vi "校准任务流程.vi"(9 "校准任务":T1[](array[typedef]), 10 "精度":dbl=4.0, 11 "模型":enum32{"线性", "多项式", "折线"}(ring)) -> ()   [LabVIEW 2016, in "斯坦道CODMn新电路板.lvlib"]
uses:
  <userlib>/_OpenG.lib/array/array.llb/Remove Duplicates from 1D Array (U16)__ogtk.vi
panel:
  out "元素":T1
  out "执行列表":T2(ring)
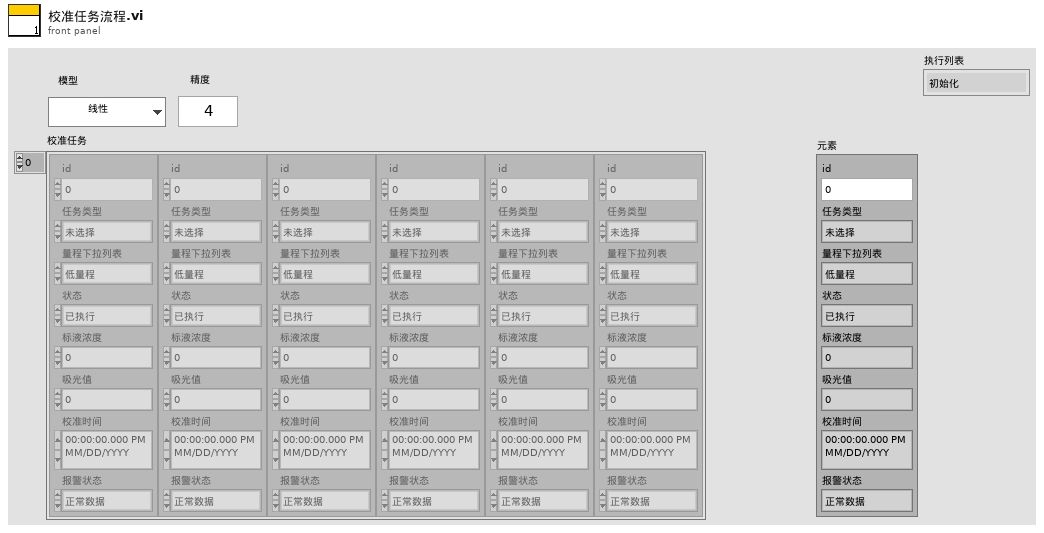
[diagram p1: front panel]
types:
  T1 = typedef "校准任务.ctl" = cluster{"id":u16, "任务类型":enum16{"未选择", "空白校准", "标样校准", "标样核查", "零点核查", "跨度核查"}, "量程下拉列表":enum16{"低量程", "高量程"}, "状态":enum16{"已执行", "待执行", "执行中", "停止"}, "标液浓度":dbl, "吸光值":dbl, "校准时间":timestamp, "报警状态":enum16{"正常数据", "报警数据"}}
  T2 = enum16{"初始化", "解析数据", "判断任务类型", "执行测试任务", "等待测试任务完成", "获取测试数据", "任务结束判定", "计算公式", "结束"}
  T3 = cluster{"时间标识":timestamp, "设备":string, "日志信息":string, "流程参数":string}
  T4 = cluster{"站号":u16, "量程切换":enum32{"H", "L", "AUTO"}, "控制命令":u16, "模式设置":enum16{"待机", "连续模式", "周期模式", "定点模式", "受控模式", "手动模式"}, "测量间隔":u16}
  T5 = cluster{"标液浓度1":dbl, "测量吸光度1":dbl, "样品1启用":bool, "标液浓度2":dbl, "测量吸光度2":dbl, "样品2启用":bool, "标液浓度3":dbl, "测量吸光度3":dbl, "样品3启用":bool, "标液浓度4":dbl, "测量吸光度4":dbl, "样品4启用":bool, "标液浓度5":dbl, "测量吸光度5":dbl, "样品5启用":bool, "模型":enum32{"线性", "多项式", "折线"}, "精度":dbl, "XY图":cluster{"X Values":dbl[], "Y Values":dbl[]}[], "拟合公式":string, "r^2":dbl, "标样一校准时间":timestamp, "标样二校准时间":timestamp, "标样三校准时间":timestamp, "标样四校准时间":timestamp, "标样五校准时间":timestamp, "二次方程":cluster{"x^2":dbl, "K":dbl, "B":dbl}, "标定时间":timestamp, "拟合公式 2":string, "r^2 2":dbl}
  T6 = enum16{"", "水样测量", "标样核查", "零点核查", "跨度核查", "空白测试", "平行样测试", "加标回收", "空白校准", "标样校准"}
  T7 = typedef "报警信息字段定义.ctl" = cluster{"时间":timestamp, "参数":string, "元器件":string, "故障现象":string, "故障分析":string, "state":string, "code":string, "platform_alarm_code":string, "是否上报":string}
  T8 = cluster{"因子编码":u32, "单位":u16, "标样参考值":sgl, "水样数据时间":timestamp, "水样实测值":sgl, "水样数据标识":string, "标样数据时间":timestamp, "标样实测值":sgl, "标样数据标识":string, "空白数据时间":timestamp, "空白实测值":sgl, "空白数据标识":string, "零点核查数据时间":timestamp, "零点核查实测值":sgl, "零点核查数据标识":string, "跨度核查数据时间":timestamp, "跨度核查实测值":sgl, "跨度核查数据标识":string, "加标回收数据时间":timestamp, "加标回收实测值":sgl, "加标回收数据标识":string, "平行样数据时间":timestamp, "平行样实测值":sgl, "平行样数据标识":string, "F0":sgl, "F1":sgl, "F2":sgl, "F3":sgl, "F4":sgl, "F5":sgl, "F6":sgl, "F7":sgl, "温度":sgl, "湿度":sgl, "X值":sgl, "fidrange":u16}
  T9 = cluster{"系统时间":timestamp, "工作状态":u16, "测量模式":enum16{"待机", "连续模式", "周期模式", "定点模式", "受控模式", "手动模式"}, "告警代码":u16, "故障代码":u16, "日志代码":u16, "软件版本":u16, "A":sgl, "B":sgl, "K":sgl, "当前滴定数":sgl, "T":sgl, "H":sgl, "id":u16, "flowid":u16, "量程":u16, "加热实时温度":sgl, "当前ORP值":sgl, "运行时间":sgl, "当前步骤剩余时间":sgl, "结束滴定数":sgl, "注射泵保温温度":sgl, "匹配滴定数X0":u16, "X^2":sgl, "X":sgl, "B 2":sgl, "光值1":sgl, "光值2":sgl, "光值3":sgl, "光值4":sgl, "光值5":sgl, "光值6":sgl, "光值7":sgl, "光值8":sgl}
  T10 = enum16{"未选择", "空白校准", "标样校准", "标样核查", "零点核查", "跨度核查"}
  T11 = cluster{"标液浓度1":dbl, "测量吸光度1":dbl, "样品1启用":bool, "标液浓度2":dbl, "测量吸光度2":dbl, "样品2启用":bool, "标液浓度3":dbl, "测量吸光度3":dbl, "样品3启用":bool, "标液浓度4":dbl, "测量吸光度4":dbl, "样品4启用":bool, "标液浓度5":dbl, "测量吸光度5":dbl, "样品5启用":bool, "模型":enum32{"线性", "多项式", "折线"}, "精度":dbl, "XY图":cluster{"X Values":dbl[], "Y Values":dbl[]}[], "拟合公式":string, "r^2":dbl, "标样一校准时间":timestamp, "标样二校准时间":timestamp, "标样三校准时间":timestamp, "标样四校准时间":timestamp, "标样五校准时间":timestamp, "二次方程":cluster{"c":dbl, "x":dbl, "x^2":dbl}, "标定时间":timestamp, "拟合公式 2":string, "r^2 2":dbl}[][]
  T12 = cluster{"标液浓度1":dbl, "测量吸光度1":dbl, "样品1启用":bool, "标液浓度2":dbl, "测量吸光度2":dbl, "样品2启用":bool, "标液浓度3":dbl, "测量吸光度3":dbl, "样品3启用":bool, "标液浓度4":dbl, "测量吸光度4":dbl, "样品4启用":bool, "标液浓度5":dbl, "测量吸光度5":dbl, "样品5启用":bool, "模型":enum32{"线性", "多项式", "折线"}, "精度":dbl, "XY图":cluster{"X Values":dbl[], "Y Values":dbl[]}[], "拟合公式":string, "r^2":dbl, "标样一校准时间":timestamp, "标样二校准时间":timestamp, "标样三校准时间":timestamp, "标样四校准时间":timestamp, "标样五校准时间":timestamp, "二次方程":cluster{"c":dbl, "x":dbl, "x^2":dbl}, "标定时间":timestamp, "拟合公式 2":string, "r^2 2":dbl}
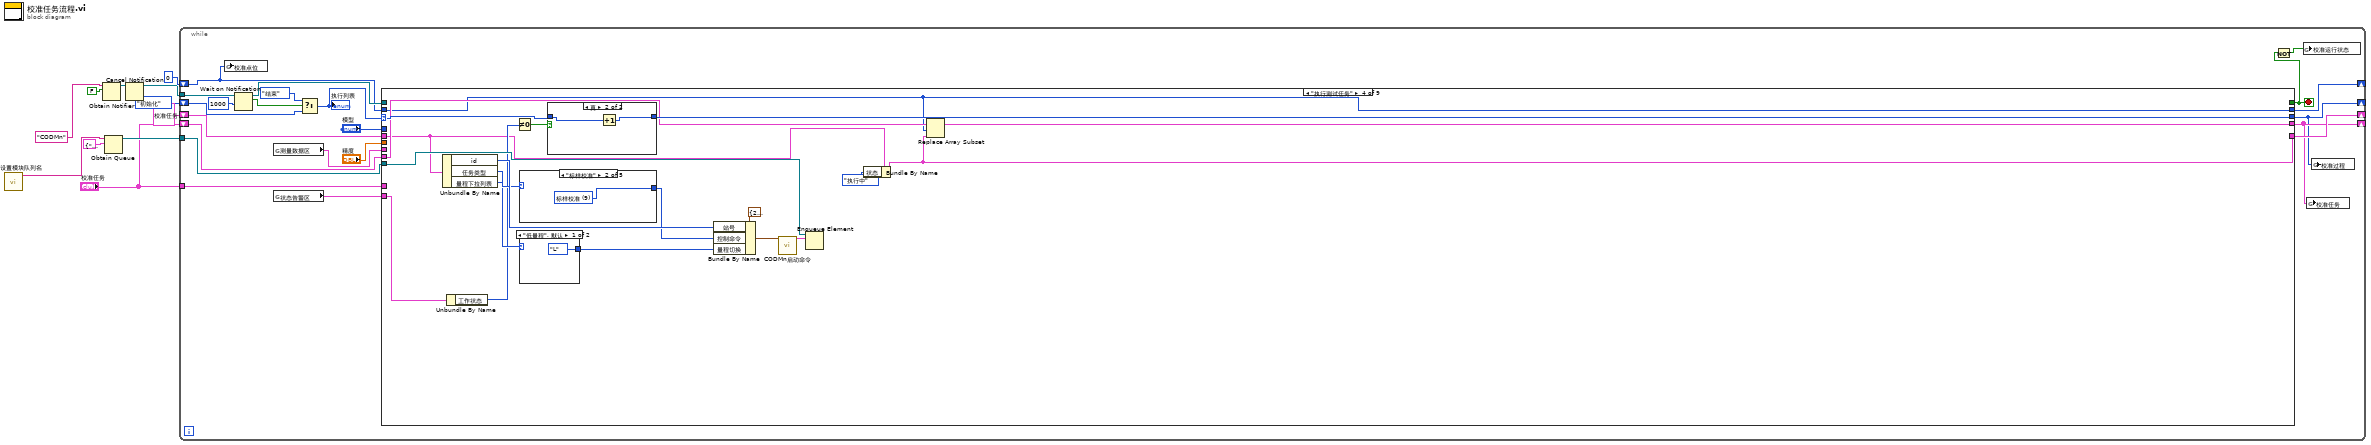
[diagram p0: block diagram]
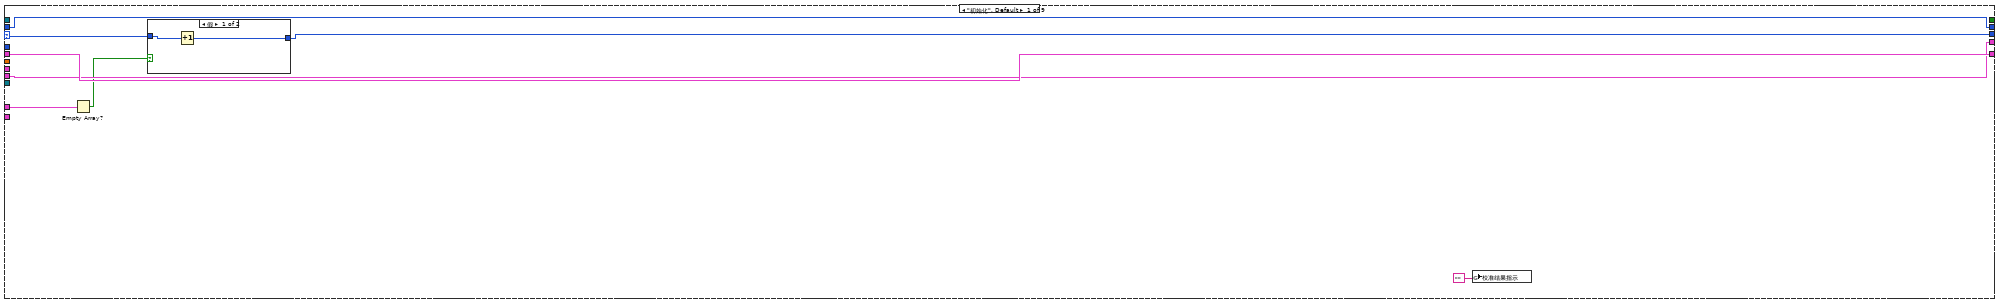
[diagram p2: hidden frame]
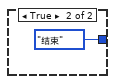
[diagram p3: hidden frame]
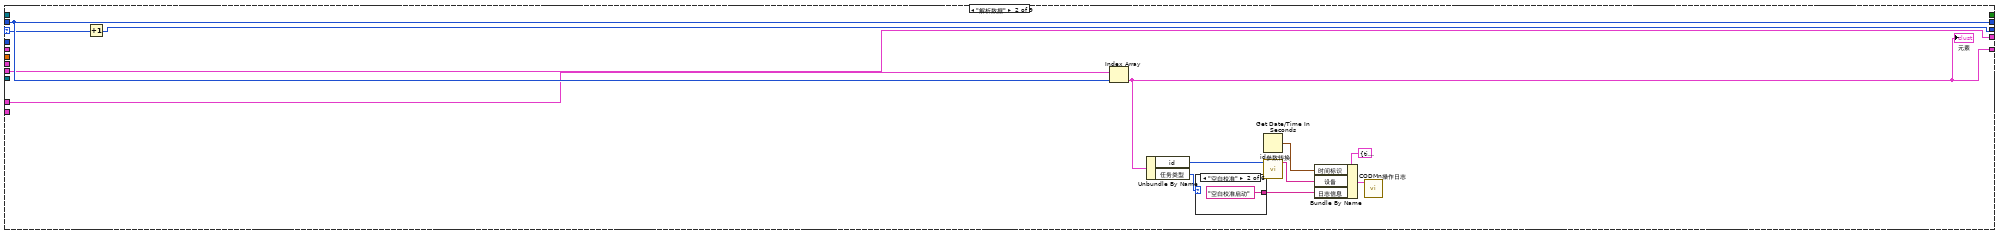
[diagram p4: hidden frame]
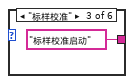
[diagram p6: hidden frame]
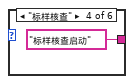
[diagram p7: hidden frame]
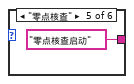
[diagram p8: hidden frame]
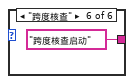
[diagram p9: hidden frame]
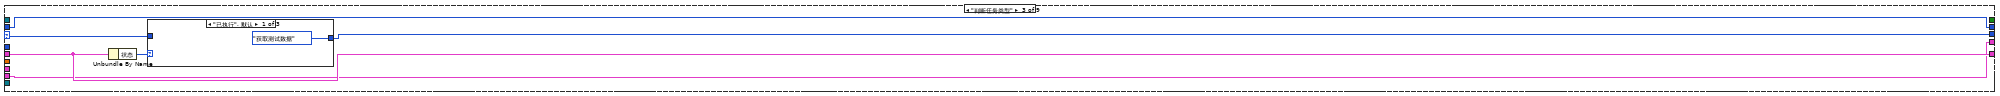
[diagram p10: hidden frame]
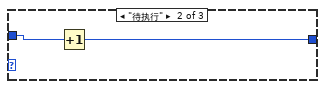
[diagram p11: hidden frame]
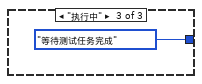
[diagram p12: hidden frame]
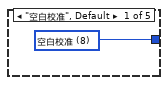
[diagram p14: hidden frame]
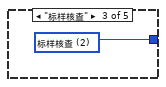
[diagram p15: hidden frame]
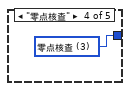
[diagram p16: hidden frame]
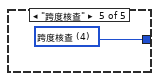
[diagram p17: hidden frame]
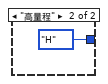
[diagram p18: hidden frame]
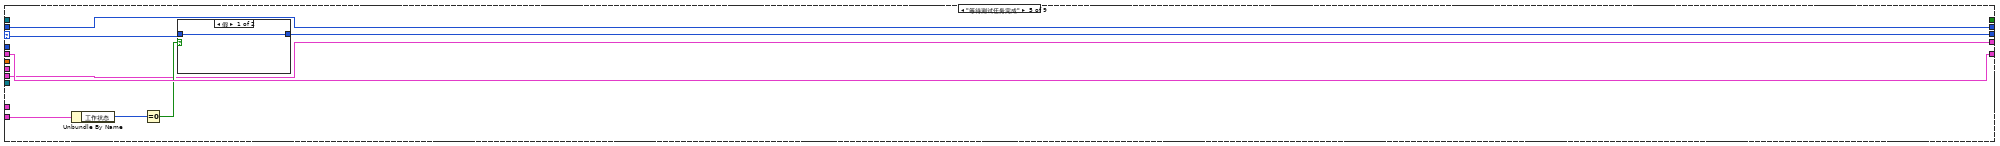
[diagram p19: hidden frame]
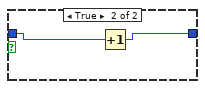
[diagram p20: hidden frame]
diagram:
  n1 = call "设置模块队列名.vi"() -> ("Msg"=w1:string)  [unwired: 11 in]
  n2 = Obtain Notifier(name (unnamed)="CODMn" ("名称（未命名）"), notification data type=FALSE) -> (notifier out=w6:refnum<notifier>)  [unwired: 2 in, 2 out]
  n3 = Obtain Queue(name (unnamed)=w1, element data type=cluster{"命令":string, "data":variant} {"命令"="", "data"=variant}) -> (queue out=w7:refnum<queue>)  [unwired: 3 in, 2 out]
  n4 = Cancel Notification(0:w6) -> (8:w5:refnum<notifier>)  [unwired: 1 in, 2 out]
  n5 = while {
    shift-right: [w13] -> _
    shift-left: 0 -> [w15]
    shift-right: [w33] -> _
    shift-left: T1 {"id"=0, "任务类型"=enum."未选择", "量程下拉列表"=enum."低量程", "状态"=enum."待执行", "标液浓度"=0.0, "吸光值"=0.0, "校准时间"=timestamp(0 s since 1904-01-01), "报警状态"=enum."正常数据"} ("校准任务") -> [w32]
    shift-right: [w12] -> _
    shift-left: T2."初始化" ("执行列表") -> [w21]
    tunnel: w7 -> [w31]
    tunnel: w5 -> [w30]
    tunnel: "校准任务" -> [w27]
    shift-right: [w14] -> _
    shift-left: "校准任务" -> [w26]
    stop <- w16 stop-if-true
    n6 = global write "VARCODMn全局变量.vi" "校准点位"(w15) -> ()
    n7 = Wait on Notification(notifier=w30, timeout in ms (-1)=1000 ("超时毫秒(-1)")) -> (notifier out=w23:refnum<notifier>, notification=w22:bool)  [unwired: 2 in, 2 out]
    n8 = global read "VARCODMn全局变量.vi" "测量数据区"() -> (w28:T8)
    n9 = global read "VARCODMn全局变量.vi" "状态告警区"() -> (w29:T9)
    n10 = Select(t=T2."结束", s=w22, f=w21) -> (s? t:f=w20:T2)
    "执行列表" <- w20
    n11 = case shown="\"执行测试任务\"" w20 {
      selector: w20 -> [w39 w56 w65 w83 w106 w124 w167 w181 w375]
      tunnel: w15 -> [w40 w57 w67 w79 w109 w115 w168 w179 w373]
      tunnel: [w41 w48 w68 w76 w110 w119 w169 w178 w374] -> w33
      tunnel: w32 -> [w41 _ w68 w78 w110 w119 w169 w178 w374]
      tunnel: [w40 w57 w67 w79 w109 w115 w164 w179 w373] -> w13
      tunnel: [_ _ _ _ _ _ _ _ TRUE] -> w16
      tunnel: [w38 w55 w64 w82 w104 w123 w166 w180 w375] -> w12
      tunnel: w31 -> [_ _ _ w91 _ _ _ _ w370]
      tunnel: w23 -> [_ _ _ _ _ _ _ _ w369]
      tunnel: w29 -> [_ _ _ w86 w108 w114 _ _ _]
      tunnel: w28 -> [_ _ _ _ _ w126 _ _ _]
      tunnel: w27 -> [w36 w54 _ _ _ _ w165 _ _]
      tunnel: [w35 w53 w63 w80 w103 w121 w161 w177 w371] -> w14
      tunnel: w26 -> [w35 w53 w63 w81 w103 w120 w161 w177 w371]
      tunnel: "模型" -> [_ _ _ _ _ _ _ w176 _]
      tunnel: "精度" -> [_ _ _ _ _ _ _ w175 _]
      frame "初始化", Default {
        n12 = Empty Array?(array=w36) -> (empty?=w34:bool)
        n13 = case shown="假" w34 {
          tunnel: w39 -> [w43 _]
          tunnel: [w42 T2."结束"] -> w38
          frame False {
            n14 = Increment(x=w43) -> (x+1=w42:T2)
          }
          frame True {
          }
        }
        n15 = global write "VARCODMn全局变量.vi" "校准结果指示"("") -> ()
      }
      frame "解析数据" {
        n16 = Increment(x=w56) -> (x+1=w55:T2)
        n17 = Index Array(array=w54, index=w57) -> (element=w48:T1)
        "元素" <- w48
        n18 = Unbundle By Name(w48) -> ("id"=w47:u16, "任务类型"=w46:T10)
        n19 = case shown="\"空白校准\"" w46 {
          tunnel: [_ "空白校准启动" "标样校准启动" "标样核查启动" "零点核查启动" "跨度核查启动"] -> w45
          frame "未选择", Default {
          }
          frame "空白校准" {
          }
          frame "标样校准" {
          }
          frame "标样核查" {
          }
          frame "零点核查" {
          }
          frame "跨度核查" {
          }
        }
        n20 = Get Date/Time In Seconds() -> (seconds since 1Jan1904=w52:timestamp)
        n21 = call "id参数转换.vi"("id"=w47) -> ("table输出"=w49:string)  [unwired: 10 in]
        n22 = Bundle By Name(cluster=T3 {"时间标识"=timestamp(0 s since 1904-01-01), "设备"="", "日志信息"="", "流程参数"=""} ("data in"), "时间标识"=w52, "设备"=w49, "日志信息"=w45) -> (w51:T3)
        n23 = call "CODMn操作日志.vi"("data in"=w51) -> ()  [unwired: 11 in]
      }
      frame "判断任务类型" {
        n24 = Unbundle By Name(w68) -> ("状态"=w66:enum16{"已执行", "待执行", "执行中", "停止"})
        n25 = case shown="\"已执行\", 默认" w66 {
          tunnel: w65 -> [_ w71 _]
          tunnel: [T2."获取测试数据" w70 T2."等待测试任务完成"] -> w64
          frame "已执行", Default {
          }
          frame "待执行" {
            n26 = Increment(x=w71) -> (x+1=w70:T2)
          }
          frame "执行中" {
          }
        }
      }
      frame "执行测试任务" {
        n27 = Unbundle By Name(w78) -> ("id"=w90:u16, "任务类型"=w89:T10, "量程下拉列表"=w88:enum16{"低量程", "高量程"})
        n28 = Unbundle By Name(w86) -> ("工作状态"=w85:u16)
        n29 = Not Equal To 0?(x=w85) -> (x != 0?=w84:bool)
        n30 = case shown="\"标样校准\"" w89 {
          tunnel: [w96 w97 w98 w99 w100] -> w73
          frame "空白校准", Default {
            w96 = u16 8 items=["启动测量"=1, "标样核查"=2, "零点核查"=3, "跨度核查"=4, "空白测试"=5, "平行样测试"=6, "加标回收"=7, "空白校准"=8, "标样校准"=9, "初始化（清洗）"=10, "停止测试"=11, "仪器重启"=12, "校时"=13, "模式设置"=14, "测量间隔设置"=15, "调试"=22, "填充管路"=30, "清洗管路"=31, "清洗反应杯"=32] ("控制命令")
          }
          frame "标样校准" {
            w97 = u16 9 items=["启动测量"=1, "标样核查"=2, "零点核查"=3, "跨度核查"=4, "空白测试"=5, "平行样测试"=6, "加标回收"=7, "空白校准"=8, "标样校准"=9, "初始化（清洗）"=10, "停止测试"=11, "仪器重启"=12, "校时"=13, "模式设置"=14, "测量间隔设置"=15, "调试"=22, "填充管路"=30, "清洗管路"=31, "清洗反应杯"=32] ("控制命令")
          }
          frame "标样核查" {
            w98 = u16 2 items=["启动测量"=1, "标样核查"=2, "零点核查"=3, "跨度核查"=4, "空白测试"=5, "平行样测试"=6, "加标回收"=7, "空白校准"=8, "标样校准"=9, "初始化（清洗）"=10, "停止测试"=11, "仪器重启"=12, "校时"=13, "模式设置"=14, "测量间隔设置"=15, "调试"=22, "填充管路"=30, "清洗管路"=31, "清洗反应杯"=32] ("控制命令")
          }
          frame "零点核查" {
            w99 = u16 3 items=["启动测量"=1, "标样核查"=2, "零点核查"=3, "跨度核查"=4, "空白测试"=5, "平行样测试"=6, "加标回收"=7, "空白校准"=8, "标样校准"=9, "初始化（清洗）"=10, "停止测试"=11, "仪器重启"=12, "校时"=13, "模式设置"=14, "测量间隔设置"=15, "调试"=22, "填充管路"=30, "清洗管路"=31, "清洗反应杯"=32] ("控制命令")
          }
          frame "跨度核查" {
            w100 = u16 4 items=["启动测量"=1, "标样核查"=2, "零点核查"=3, "跨度核查"=4, "空白测试"=5, "平行样测试"=6, "加标回收"=7, "空白校准"=8, "标样校准"=9, "初始化（清洗）"=10, "停止测试"=11, "仪器重启"=12, "校时"=13, "模式设置"=14, "测量间隔设置"=15, "调试"=22, "填充管路"=30, "清洗管路"=31, "清洗反应杯"=32] ("控制命令")
          }
        }
        n31 = case shown="\"低量程\", 默认" w88 {
          tunnel: [enum32{"H", "L", "AUTO"}."L" ("量程切换") enum32{"H", "L", "AUTO"}."H" ("量程切换")] -> w87
          frame "低量程", Default {
          }
          frame "高量程" {
          }
        }
        n32 = case shown="真" w84 {
          tunnel: w83 -> [w93 w95]
          tunnel: [w93 w94] -> w82
          frame False {
          }
          frame True {
            n33 = Increment(x=w95) -> (x+1=w94:T2)
          }
        }
        n34 = Bundle By Name(cluster=T4 {"站号"=21, "量程切换"=enum."AUTO", "控制命令"=0, "模式设置"=enum."待机", "测量间隔"=0} ("参数"), "站号"=w90, "控制命令"=w73, "量程切换"=w87) -> (w74:T4)
        n35 = call "CODMn启动命令.vi"("参数"=w74) -> ("启动命令"=w92:cluster{"命令":string, "data":variant})  [unwired: 10 in]
        n36 = Enqueue Element(queue=w91, element=w92) -> ()  [unwired: 2 in, 3 out]
        n37 = Bundle By Name(cluster=w78, "状态"=enum16{"已执行", "待执行", "执行中", "停止"}."执行中") -> (w76:T1)
        n38 = Replace Array Subset(array=w81, new element=w76, index=w79) -> (w80:T1[])
      }
      frame "等待测试任务完成" {
        n39 = Unbundle By Name(w108) -> ("工作状态"=w107:u16)
        n40 = Equal To 0?(x=w107) -> (x = 0?=w105:bool)
        n41 = case shown="假" w105 {
          tunnel: w106 -> [w111 w113]
          tunnel: [w111 w112] -> w104
          frame False {
          }
          frame True {
            n42 = Increment(x=w113) -> (x+1=w112:T2)
          }
        }
      }
      frame "获取测试数据" {
        n43 = Unbundle By Name(w119) -> ("任务类型"=w125:T10, "状态"=w118:enum16{"已执行", "待执行", "执行中", "停止"})
        n44 = Increment(x=w124) -> (x+1=w123:T2)
        n45 = case shown="\"待执行\", 默认" w118 {
          tunnel: w126 -> [_ w135]
          tunnel: w125 -> [_ w134]
          tunnel: [w127 w131] -> w122
          tunnel: w119 -> [w127 w130]
          tunnel: w114 -> [_ w129]
          frame "已执行" {
          }
          frame "待执行", Default {
            n46 = case shown="\"跨度核查\"" w134 {
              tunnel: w135 -> [w140 w145 w150 w155 w160]
              tunnel: [w139 w144 w149 w154 w159] -> w132
              tunnel: [w137 w142 w147 w152 w157] -> w133
              tunnel: w129 -> [w138 w143 w148 w153 w158]
              tunnel: [w136 w141 w146 w151 w156] -> w128
              frame "空白校准", Default {
                n47 = Unbundle By Name(w138) -> ("结束滴定数"=w137:sgl, "告警代码"=w136:u16)
                n48 = Unbundle By Name(w140) -> ("空白数据时间"=w139:timestamp)
              }
              frame "标样校准" {
                n49 = Unbundle By Name(w143) -> ("结束滴定数"=w142:sgl, "告警代码"=w141:u16)
                n50 = Unbundle By Name(w145) -> ("标样数据时间"=w144:timestamp)
              }
              frame "标样核查" {
                n51 = Unbundle By Name(w148) -> ("结束滴定数"=w147:sgl, "告警代码"=w146:u16)
                n52 = Unbundle By Name(w150) -> ("标样数据时间"=w149:timestamp)
              }
              frame "零点核查" {
                n53 = Unbundle By Name(w155) -> ("零点核查数据时间"=w154:timestamp)
                n54 = Unbundle By Name(w153) -> ("结束滴定数"=w152:sgl, "告警代码"=w151:u16)
              }
              frame "跨度核查" {
                n55 = Unbundle By Name(w158) -> ("结束滴定数"=w157:sgl, "告警代码"=w156:u16)
                n56 = Unbundle By Name(w160) -> ("跨度核查数据时间"=w159:timestamp)
              }
            }
            n57 = Bundle By Name(cluster=w130, "校准时间"=w132, "吸光值"=w133, "报警状态"=w128) -> (w131:T1)
          }
        }
        n58 = Bundle By Name(cluster=w122, "状态"=enum16{"已执行", "待执行", "执行中", "停止"}."已执行") -> (w116:T1)
        n59 = Replace Array Subset(array=w120, new element=w116, index=w115) -> (w121:T1[])
      }
      frame "任务结束判定" {
        n60 = Array Size(array=w165) -> (size(s)=w163:i32)
        n61 = Increment(x=w168) -> (x+1=w164:i32)
        n62 = Greater Or Equal?(x=w164, y=w163) -> (x >= y?=w162:bool)
        n63 = case shown="假" w162 {
          tunnel: w167 -> [_ w173]
          tunnel: [T2."解析数据" w172] -> w166
          frame False {
            n64 = Wait (ms)(milliseconds to wait=u32 3000 ("等待时间（毫秒）")) -> ()  [unwired: 1 out]
          }
          frame True {
            n65 = Increment(x=w173) -> (x+1=w172:T2)
          }
        }
      }
      frame "计算公式" {
        n66 = flat-sequence {
          tunnel: w181 -> [w188]
          tunnel: w177 -> [w184]
          tunnel: w176 -> [w183]
          tunnel: w175 -> [w182]
          tunnel: [w187] -> w174
          tunnel: [w368] -> w180
          tunnel: w174 -> [w368]
          frame #0 {
            n67 = for {
              tunnel: w184 -> [w367] mode=indexing
              tunnel: [w366] -> w186 mode=indexing
              n68 = Unbundle By Name(w367) -> ("id"=w366:u16)
            }
            n69 = Increment(x=w188) -> (x+1=w187:T2)
            n70 = call-poly <userlib>:"Remove Duplicates from 1D Array__ogtk.vi"("Input Array"=w186) -> ("Output Array"=w185:u16[])  [unwired: 1 out]
            n71 = for {
              tunnel: w185 -> [w201] mode=indexing
              tunnel: w184 -> [w203]
              tunnel: w183 -> [w200]
              tunnel: w182 -> [w199]
              n72 = for {
                tunnel: w203 -> [w363] mode=indexing
                tunnel: w201 -> [w365]
                tunnel: [w363] -> w202 mode=indexing if=w364
                n73 = Unbundle By Name(w363) -> ("id"=w362:u16)
                n74 = Equal?(x=w362, y=w365) -> (x = y?=w364:bool)
              }
              n75 = flat-sequence {
                tunnel: w202 -> [w216]
                tunnel: w201 -> [w211]
                tunnel: w200 -> [w215]
                tunnel: w199 -> [w214]
                tunnel: T5 {"标液浓度1"=0.0, "测量吸光度1"=0.0, "样品1启用"=FALSE, "标液浓度2"=0.0, "测量吸光度2"=0.0, "样品2启用"=FALSE, "标液浓度3"=0.0, "测量吸光度3"=0.0, "样品3启用"=FALSE, "标液浓度4"=0.0, "测量吸光度4"=0.0, "样品4启用"=FALSE, "标液浓度5"=0.0, "测量吸光度5"=0.0, "样品5启用"=FALSE, "模型"=enum."线性", "精度"=4.0, "XY图"=[], "拟合公式"="", "r^2"=0.0, "标样一校准时间"=timestamp(0 s since 1904-01-01), "标样二校准时间"=timestamp(0 s since 1904-01-01), "标样三校准时间"=timestamp(0 s since 1904-01-01), "标样四校准时间"=timestamp(0 s since 1904-01-01), "标样五校准时间"=timestamp(0 s since 1904-01-01), "二次方程"={"x^2"=0.0, "K"=0.0, "B"=0.0}, "标定时间"=timestamp(0 s since 1904-01-01), "拟合公式 2"="", "r^2 2"=0.0} ("曲线模型") -> [w213]
                tunnel: [w212] -> w198
                tunnel: [w211] -> w197
                tunnel: [w210] -> w196
                tunnel: [w209] -> w194
                tunnel: cluster{"x^2":dbl, "K":dbl, "B":dbl} {"x^2"=0.0, "K"=0.0, "B"=0.0} ("二次方程 2") -> [w208]
                tunnel: [w207] -> w193
                tunnel: 0.0 ("公式切换阈值滴定数(0~9999)") -> [w206]
                tunnel: [w205] -> w191
                tunnel: TRUE -> [w204]
                tunnel: w198 -> [w290]
                tunnel: w197 -> [w292]
                tunnel: w196 -> [w291]
                tunnel: w194 -> [w288]
                tunnel: w193 -> [w287]
                tunnel: w191 -> [w282]
                frame #0 {
                  n76 = for {
                    tunnel: w216 -> [w238] mode=indexing
                    tunnel: w211 -> [_]
                    tunnel: w215 -> [w235]
                    tunnel: w214 -> [w234]
                    shift-right: [w226] -> w212
                    shift-left: w213 -> [w233]
                    tunnel: [w224] -> w210
                    shift-right: [w223] -> w209
                    shift-left: w208 -> [_]
                    shift-right: [w222] -> w207
                    shift-left: w206 -> [_]
                    shift-right: [w219] -> w205
                    shift-left: w204 -> [w217]
                    n77 = Unbundle By Name(w238) -> ("标液浓度"=w237:dbl, "吸光值"=w236:dbl, "任务类型"=w225:T10, "量程下拉列表"=w224:enum16{"低量程", "高量程"}, "校准时间"=w232:timestamp, "报警状态"=w220:enum16{"正常数据", "报警数据"})
                    n78 = Get Date/Time In Seconds() -> (seconds since 1Jan1904=w228:timestamp)
                    n79 = Greater Than 0?(x=w220) -> (x > 0?=w218:bool)
                    n80 = case shown="假" w218 {
                      tunnel: [w239 FALSE] -> w219
                      tunnel: w217 -> [w239 _]
                      frame False {
                      }
                      frame True {
                      }
                    }
                    n81 = case shown="\"空白校准\"" w225 {
                      tunnel: w237 -> [_ w249 w257 w265 w273 w281]
                      tunnel: w236 -> [_ w248 w250 w264 w272 w280]
                      tunnel: w235 -> [_ w247 w256 w263 w271 w279]
                      tunnel: w234 -> [_ w246 w255 w262 w270 w278]
                      tunnel: w233 -> [w241 w244 w253 w260 w268 w276]
                      tunnel: [w241 w242 w252 w259 w267 w275] -> w231
                      tunnel: w232 -> [_ w243 w251 w258 w266 w274]
                      frame "未选择", Default {
                        (unwired) T6."" ("测量模式")
                      }
                      frame "空白校准" {
                        n82 = Bundle By Name(cluster=w244, "标液浓度1"=w249, "测量吸光度1"=w248, "模型"=w247, "精度"=w246, "样品1启用"=TRUE, "标样一校准时间"=w243) -> (w242:T5)
                      }
                      frame "标样校准" {
                        (unwired) T6."标样校准" ("测量模式")
                        n83 = Bundle By Name(cluster=w253, "标液浓度2"=w257, "测量吸光度2"=w250, "模型"=w256, "精度"=w255, "样品2启用"=TRUE ("样品1启用"), "标样二校准时间"=w251) -> (w252:T5)
                      }
                      frame "标样核查" {
                        (unwired) T6."标样核查" ("测量模式")
                        n84 = Bundle By Name(cluster=w260, "标液浓度3"=w265, "测量吸光度3"=w264, "模型"=w263, "精度"=w262, "样品3启用"=TRUE ("样品1启用"), "标样三校准时间"=w258) -> (w259:T5)
                      }
                      frame "零点核查" {
                        (unwired) T6."零点核查" ("测量模式")
                        n85 = Bundle By Name(cluster=w268, "标液浓度4"=w273, "测量吸光度4"=w272, "模型"=w271, "精度"=w270, "样品4启用"=TRUE ("样品1启用"), "标样四校准时间"=w266) -> (w267:T5)
                      }
                      frame "跨度核查" {
                        (unwired) T6."跨度核查" ("测量模式")
                        n86 = Bundle By Name(cluster=w276, "标液浓度5"=w281, "测量吸光度5"=w280, "模型"=w279, "精度"=w278, "样品5启用"=TRUE ("样品1启用"), "标样五校准时间"=w274) -> (w275:T5)
                      }
                    }
                    n87 = global read "校准数据全局变量.vi" "CODMn曲线模型"() -> (w230:T11)
                    n88 = call "曲线模型计算.vi"("曲线模型"=w231) -> ("公式切换阈值滴定数(0~9999)"=w222:dbl, "二次方程 2"=w223:cluster{"x^2":dbl, "K":dbl, "B":dbl}, "输出簇"=w227:T12)  [unwired: 8 in]
                    n89 = Bundle By Name(cluster=w227, "标定时间"=w228) -> (w226:T12)
                    n90 = Replace Array Subset(array=w230, new element=w226, index (row)=T6."水样测量" ("测量模式"), index (col)=w224) -> (w229:T11)
                    n91 = global write "校准数据全局变量.vi" "CODMn曲线模型"(w229) -> ()
                  }
                }
                frame #1 {
                  n92 = Unbundle By Name(w290) -> ("r^2"=w285:dbl, "r^2 2"=w284:dbl, "二次方程"=w293:cluster{"x^2":dbl, "K":dbl, "B":dbl}, "模型"=w286:enum32{"线性", "多项式", "折线"})
                  n93 = case shown="\"线性\", 默认" w286 {
                    tunnel: w285 -> [w298 w302]
                    tunnel: w284 -> [_ w303]
                    tunnel: [w295 w304] -> w283
                    tunnel: w282 -> [w294 w300]
                    frame "线性", Default {
                      n94 = global read "CODMn断电保存全局变量.vi" "校准条件"() -> (w299:cluster{"线性相关系数":dbl})
                      n95 = Unbundle By Name(w299) -> ("线性相关系数"=w297:dbl)
                      n96 = Greater Or Equal?(x=w298, y=w297) -> (x >= y?=w296:bool)
                      n97 = And(x=w294, y=w296) -> (x .and. y?=w295:bool)
                    }
                    frame "折线" {
                      n98 = global read "CODMn断电保存全局变量.vi" "校准条件"() -> (w307:cluster{"线性相关系数":dbl})
                      n99 = Unbundle By Name(w307) -> ("线性相关系数"=w301:dbl)
                      n100 = Greater Or Equal?(x=w302, y=w301) -> (x >= y?=w306:bool)
                      n101 = Greater Or Equal?(x=w303, y=w301) -> (x >= y?=w305:bool)
                      n102 = Compound Arithmetic op=AND ("复合运算")(w306, w305, w300) -> (w304:bool)
                    }
                  }
                  n103 = case shown="真" w283 {
                    tunnel: w293 -> [_ w332]
                    tunnel: w292 -> [w313 _]
                    tunnel: w291 -> [_ w321]
                    tunnel: w290 -> [_ w331]
                    tunnel: [w308 w330] -> w289
                    tunnel: w288 -> [_ w329]
                    tunnel: w287 -> [_ w320]
                    tunnel: w282 -> [w310 _]
                    frame False {
                      n104 = case shown="假" w310 {
                        tunnel: ["有故障数据" ("格式字符串") "校准条件未满足" ("格式字符串")] -> w309
                        frame False {
                        }
                        frame True {
                        }
                      }
                      n105 = call "id参数转换.vi"("id"=w313) -> ("table输出"=w312:string)  [unwired: 10 in]
                      n106 = Get Date/Time In Seconds() -> (seconds since 1Jan1904=w316:timestamp)
                      n107 = Format Into String(format string="校准失败，%s" ("格式字符串"), w309) -> (resulting string=w308:string)  [unwired: 2 in, 1 out]
                      n108 = Bundle By Name(cluster=T3 {"时间标识"=timestamp(0 s since 1904-01-01), "设备"="", "日志信息"="", "流程参数"=""} ("data in"), "时间标识"=w316, "设备"=w312, "日志信息"=w308) -> (w315:T3)
                      n109 = call "CODMn操作日志.vi"("data in"=w315) -> ()  [unwired: 11 in]
                    }
                    frame True {
                      n110 = Unbundle By Name(w329) -> ("x^2"=w325:dbl, "K"=w324:dbl, "B"=w323:dbl)
                      n111 = Unbundle By Name(w332) -> ("x^2"=w334:dbl, "K"=w335:dbl, "B"=w336:dbl)
                      n112 = Bundle By Name(cluster=cluster{"X^2":dbl, "X":dbl, "b":dbl} {"X^2"=0.0, "X"=0.0, "b"=0.0} ("公式"), "X^2"=w334, "X"=w335, "b"=w336) -> (w327:cluster{"X^2":dbl, "X":dbl, "b":dbl})
                      n113 = Bundle By Name(cluster=cluster{"X^2":dbl, "X":dbl, "b":dbl} {"X^2"=0.0, "X"=0.0, "b"=0.0} ("公式"), "X^2"=w325, "X"=w324, "b"=w323) -> (w322:cluster{"X^2":dbl, "X":dbl, "b":dbl})
                      n114 = for {
                        N: 7 -> [_]
                        tunnel: w327 -> [w347]
                        tunnel: [w345] -> w319
                        tunnel: w322 -> [w344]
                        tunnel: w320 -> [w343]
                        tunnel: w321 -> [w341]
                        i -> [w338]
                        w342 = enum16{"CODMn"}."CODMn" ("测量参数")
                        n115 = case shown="\"高量程\"" w341 {
                          tunnel: [enum16{"低量程1", "低量程2", "高量程1", "高量程2"}."低量程1" ("量程") enum16{"低量程1", "低量程2", "高量程1", "高量程2"}."高量程1" ("量程")] -> w340
                          tunnel: [enum16{"低量程1", "低量程2", "高量程1", "高量程2"}."低量程2" ("量程") enum16{"低量程1", "低量程2", "高量程1", "高量程2"}."高量程2" ("量程")] -> w339
                          frame "低量程", Default {
                          }
                          frame "高量程" {
                          }
                        }
                        n116 = Increment(x=w338) -> (x+1=w337:i32)
                        n117 = call "公式写入.vi"("临界滴定数"=w343, "公式"=w347, "error in (no error)"=errorcluster {"status"=FALSE, "code"=0, "source"=""} ("error out"), "量程"=w340, "测量模式"=w337, "测量参数"=w342) -> ("error out"=w346:errorcluster)  [unwired: 5 in]
                        n118 = call "公式写入.vi"("临界滴定数"=w343, "公式"=w344, "error in (no error)"=w346, "量程"=w339, "测量模式"=w337, "测量参数"=w342) -> ("error out"=w345:errorcluster)  [unwired: 5 in]
                      }
                      n119 = case shown="错误" w319 {
                        tunnel: w321 -> [w356 _]
                        tunnel: w331 -> [w354 _]
                        tunnel: ["校准成功" w359] -> w330
                        frame No Error {
                          n120 = call "校准记录.vi"("曲线模型"=w354, "量程"=w356, "测量模式"="所有测量模式") -> ()  [unwired: 8 in, 1 out]
                        }
                        frame Error {
                          w359 = "校准失败，公式写入异常"
                          n121 = Get Date/Time In Seconds() -> (seconds since 1Jan1904=w360:timestamp)
                          n122 = Bundle By Name(cluster=T7 {"时间"=timestamp(0 s since 1904-01-01), "参数"="", "元器件"="", "故障现象"="", "故障分析"="", "state"="", "code"="", "platform_alarm_code"="", "是否上报"=""} ("data"), "时间"=w360, "参数"="CODMn", "元器件"=w359) -> (w357:T7)
                          n123 = call "CODMn报警信息.vi"("data"=w357) -> ()  [unwired: 10 in, 1 out]
                        }
                      }
                    }
                  }
                  n124 = global write "VARCODMn全局变量.vi" "校准结果指示"(w289) -> ()
                }
              }
            }
          }
          frame #1 {
            n125 = call "校准数据写入配置文件.vi"() -> ()  [unwired: 11 in, 1 out]
          }
        }
      }
      frame "结束" {
        n126 = Release Notifier(notifier=w369) -> ()  [unwired: 2 in, 3 out]
        n127 = Release Queue(queue=w370) -> ()  [unwired: 2 in, 3 out]
      }
    }
    n128 = Not(x=w16) -> (.not. x?=w17:bool)
    n129 = global write "VARCODMn全局变量.vi" "校准运行状态"(w17) -> ()
    n130 = global write "VARCODMn全局变量.vi" "校准任务"(w14) -> ()
    n131 = global write "VARCODMn全局变量.vi" "校准过程"(w12) -> ()
  }
